vi "Basic_position_speed.vi"(8 "error in (no error)":errorcluster, 9 "Position m?":dbl, 10 "Speed m?":dbl=1.0, 11 "m?":string="m1") -> (0 "error out":errorcluster)   [LabVIEW 2017]
uses:
  IP Address.vi
  <vilib>/httpClient/LabVIEWHTTPClient.lvlib
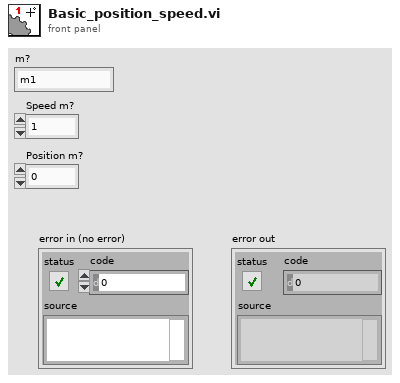
[diagram p1: front panel]
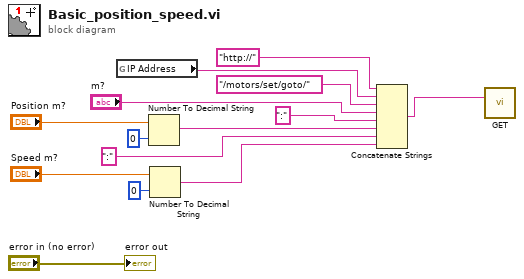
[diagram p0: block diagram]
diagram:
  n1 = global read "IP Address.vi" "IP Address"() -> (w1:string)
  n2 = Number To Decimal String(number="Position m?", width (-)=i16 0) -> (decimal integer string=w14:string)
  n3 = Number To Decimal String(number="Speed m?", width (-)=i16 0) -> (decimal integer string=w6:string)
  n4 = Concatenate Strings("http://" ("string"), w1, "/motors/set/goto/" ("url"), "m?", ":" ("string"), w14, ":" ("string"), w6) -> (w12:string)
  n5 = call <vilib>:"GET.vi"("url"=w12) -> ()  [unwired: 11 in, 4 out]
  "error out" <- "error in (no error)"
